vi "motor encoder test.vi"() -> ()   [LabVIEW 2017]
panel:
  in  "Reset":bool
  in  "stop":bool
  in  "Duty Cycle (-100 to +100)":dbl
  out "Counter Value":dbl
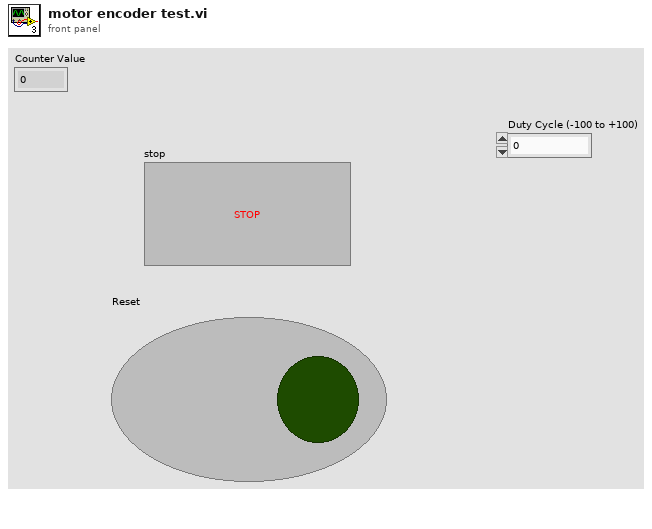
[diagram p1: front panel]
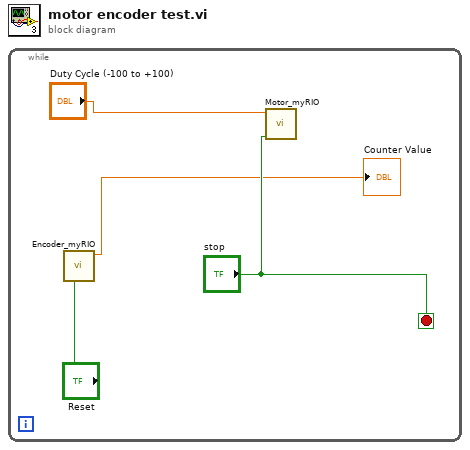
[diagram p0: block diagram]
diagram:
  n1 = while {
    stop <- "stop" stop-if-true
    n2 = call "Encoder_myRIO.vi"("Reset"="Reset") -> ("Counter Value"=→"Counter Value":dbl)  [unwired: 9 in, 1 out]
    n3 = call "Motor_myRIO.vi"("Stop VI"="stop", "Duty Cycle (-100 to +100)"="Duty Cycle (-100 to +100)") -> ()  [unwired: 10 in]
  }
